vi "Create Registered Channel Types.vi"(8 "error in":errorcluster, 11 "Channel Definition in":T1 {"Custom Config Data" format="%x"}) -> (0 "error out":errorcluster, 1 "Not Registered":bool, 2 "Channel out":refnum<class "CIFChannels.lvclass">, 3 "Channel Definition out":T1 {"Custom Config Data" format="%x"})   [LabVIEW 2021, in "ChannelRegistrar.lvlib"]
uses:
  ChannelRegistrar.lvlib
  typedef/Channel Definition.ctl
  CIFChannels/Typedef/Direction.ctl
  typedef/Registered Channel Types.ctl
  CIFChannels/CIFChannels.lvclass
  CIF_NIChn/Double/CIF_NIChn_Double.lvclass
  D:/dev/CIF-LVCore/src/Channels/CIFChannels/CIFChannels.lvclass
  CIF_NIChn/U64/CIF_NIChn_U64.lvclass
  CIF_NIChn/I64/CIF_NIChn_I64.lvclass
  CIF_NIChn/FIFO_CAN/CIF_NIChn_FifoCAN.lvclass
  CIF_NIChn/FIFO_DAQ/CIF_NIChn_Fifo_DAQ.lvclass
  D:/dev/CIF-LVCore/src/Channels/CIF_NIChn/NIChn/CIF_NIChn.lvclass
  D:/dev/CIF-LVCore/src/Channels/CIF_NIChn/Double/CIF_NIChn_Double.lvclass
  D:/dev/CIF-LVCore/src/Channels/CIF_NIChn/U64/CIF_NIChn_U64.lvclass
  D:/dev/CIF-LVCore/src/Channels/CIF_NIChn/I64/CIF_NIChn_I64.lvclass
  D:/dev/CIF-LVCore/src/Channels/CIF_NIChn/FIFO_CAN/CIF_NIChn_FifoCAN.lvclass
  D:/dev/CIF-LVCore/src/Channels/CIF_NIChn/FIFO_DAQ/CIF_NIChn_Fifo_DAQ.lvclass
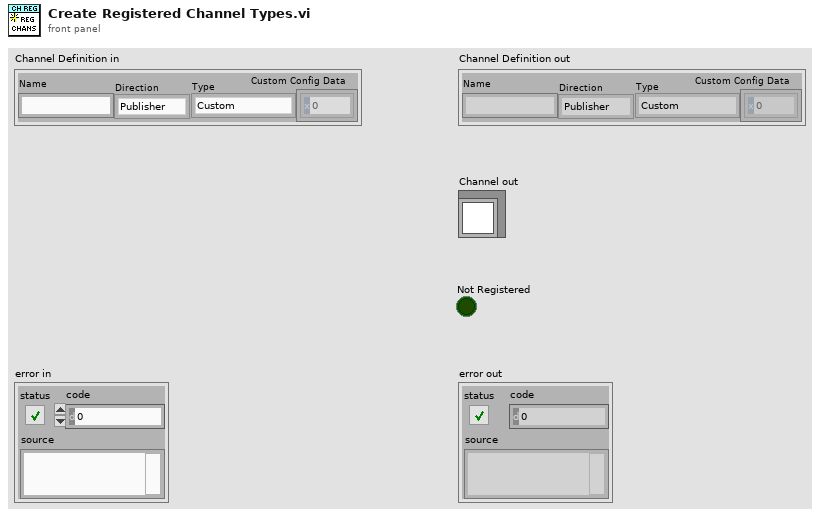
[diagram p1: front panel]
types:
  T1 = typedef "ChannelRegistrar.lvlib/Channel Definition.ctl" = cluster{"Name":string, "Direction":T2, "Type":T3, "Custom Config Data":u8[]}
  T2 = typedef "CIFChannels.lvclass/Direction.ctl" = enum16{"Publisher", "Subscriber"}
  T3 = typedef "ChannelRegistrar.lvlib/Registered Channel Types.ctl" = enum16{"Custom", "CIF_NIChn_Double", "CIF_NIChn_I64", "CIF_NIChn_U64", "CIF_NIChn_FifoCAN", "CIF_NIChn_Fifo_DAQ"}
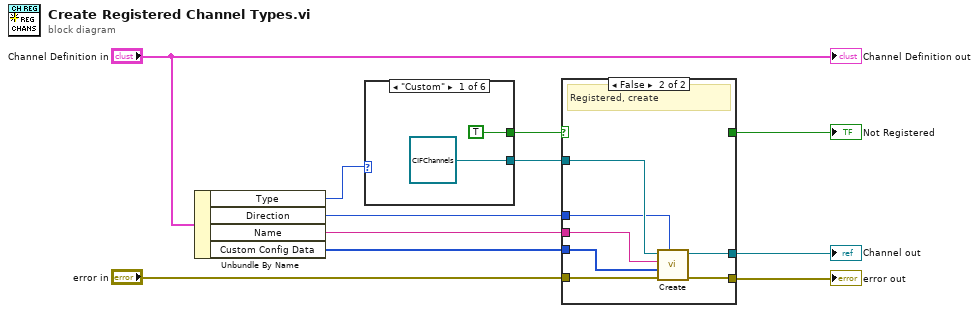
[diagram p0: block diagram]
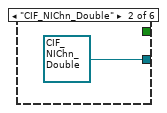
[diagram p2: hidden frame]
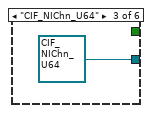
[diagram p3: hidden frame]
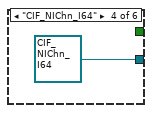
[diagram p4: hidden frame]
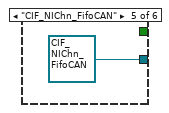
[diagram p5: hidden frame]
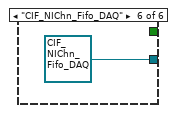
[diagram p6: hidden frame]
diagram:
  n1 = Unbundle By Name("Channel Definition in") -> ("Type"=w1:T3, "Direction"=w11:T2, "Name"=w10:string, "Custom Config Data"=w9:u8[])
  n2 = case shown="\"Custom\"" w1 {
    tunnel: [TRUE _ _ _ _ _] -> w4
    tunnel: [refnum<class "CIFChannels.lvclass"> refnum ("Channel out 2") refnum<class "CIF_NIChn_Double.lvclass"> refnum ("CIFTagDouble.lvclass") refnum<class "CIF_NIChn_U64.lvclass"> refnum ("CIFTagU64.lvclass") refnum<class "CIF_NIChn_I64.lvclass"> refnum ("CIFTagI64.lvclass") refnum<class "CIF_NIChn_FifoCAN.lvclass"> refnum ("CIFFifoCAN.lvclass") refnum<class "CIF_NIChn_Fifo_DAQ.lvclass"> refnum ("CIF_NIChn_Fifo_DAQ.lvclass")] -> w3
    frame "Custom" {
    }
    frame "CIF_NIChn_Double" {
    }
    frame "CIF_NIChn_U64" {
    }
    frame "CIF_NIChn_I64" {
    }
    frame "CIF_NIChn_FifoCAN" {
    }
    frame "CIF_NIChn_Fifo_DAQ" {
    }
  }
  n3 = case shown="False" w4 {
    selector: w4 -> [w19 _]
    tunnel: w11 -> [_ w24]
    tunnel: w10 -> [_ w23]
    tunnel: w9 -> [_ w22]
    tunnel: "error in" -> [w20 w26]
    tunnel: [w20 w25] -> w7
    tunnel: [_ w21] -> w2
    tunnel: [w19 _] -> w5
    tunnel: w3 -> [_ w27]
    frame True {
      # "Not registered"
    }
    frame False {
      # "Registered, create"
      n4 = call-dynamic "Create.vi"("Direction"=w24, "error in (no error)"=w26, "Custom Config Data"=w22, "Name"=w23, "CIFChannels in"=w27) -> ("error out"=w25:errorcluster, "CIFChannels out"=w21:refnum<class "CIFChannels.lvclass">)  [unwired: 5 in]
    }
  }
  "error out" <- w7
  "Channel out" <- w2
  "Not Registered" <- w5
  "Channel Definition out" <- "Channel Definition in"
